vi "Read Global Locked.vi"(7 "Semaphore Timeout":i32=-1, 8 "error in (no error)":errorcluster, 11 "Shifter in":refnum<class "Shifter.lvclass">) -> (0 "error out":errorcluster, 1 "Semaphore Timed Out":bool, 2 "Global":refnum<class "System.lvclass">, 3 "Shifter out":refnum<class "Shifter.lvclass">)   [LabVIEW 2013, in "Shifter.lvclass"]
uses:
  Shifter.lvclass
  System/System.lvclass
  Robot Global Data.vi
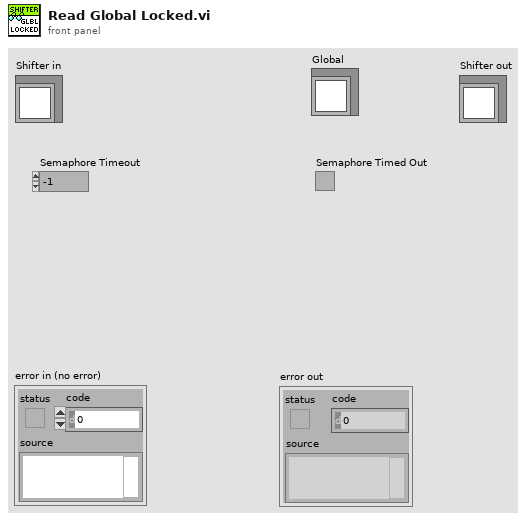
[diagram p1: front panel]
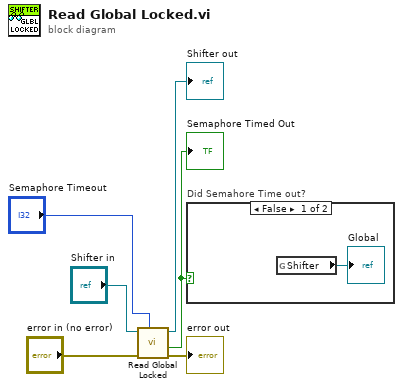
[diagram p0: block diagram]
diagram:
  n1 = call-parent "Read Global Locked.vi"("Semaphore Timeout"="Semaphore Timeout", "error in (no error)"="error in (no error)", "System in"="Shifter in") -> ("error out"=→"error out":errorcluster, "Semaphore Timed Out"=w2:bool, "System out"=→"Shifter out":refnum<class "Shifter.lvclass">)  [unwired: 5 in, 1 out]
  "Semaphore Timed Out" <- w2
  n2 = case "Did Semahore Time out?" shown="False" w2 {
    frame False {
      n3 = global read "Robot Global Data.vi" "Shifter"() -> (→"Global":refnum<class "Shifter.lvclass">)
    }
    frame True {
    }
  }
